vi "AutoDiscardBeads.vi"(10 "Minimum bead validity":dbl=1.0, 11 "Buffer Image":T1) -> ()   [LabVIEW 2011]
uses:
  <vilib>/vision/Image Controls.llb/IMAQ Image.ctl
  GlobalVariables.vi
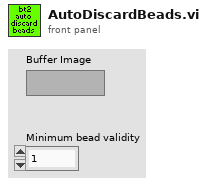
[diagram p1: front panel]
types:
  T1 = typedef "IMAQ Image.ctl" = refnum<image>
  T2 = typedef "MeasureConfigType.ctl" = cluster{"Bead locations":cluster{"X":i32, "Y":i32}[], "ROI":i32, "Experiment base path":path, "Image output subdir":string, "Output mode":T3, "Traces output subdir":string, "QTrk Settings":T4, "Tracking Config":T5, "Experiment Name":string, "Program":T8, "ZLUT":sgl[][][], "Camera settings":T15, "Experiment Script":string, "Max frames in memory":i32, "Save traces as binary":bool, "Pixel Calibration Gain Image":string, "Pixel Calibration Offset Image":string, "Use pixel calibration images":bool, "Internal camera settings":string, "Trace write interval":i32}
  T3 = typedef "MeasureConfigOutputMode.ctl" = enum16{"None", "Track", "SaveImages"}
  T4 = typedef "QTrkSettings.ctl" = cluster{"Image width":i32, "Image height":i32, "Number of threads (CPU based)":i32, "CUDA Device":i32, "COM Background correction factor":sgl, "ZLUT MinRadius":sgl, "ZLUT Radial sample density":sgl, "ZLUT Angular sample density":sgl, "ZLUT ROI Coverage":sgl, "QI Iterations":i32, "QI MinRadius":sgl, "QI Radial sample density":sgl, "QI Angular sample density":sgl, "QI ROI Coverage":sgl, "QI Angular Step \nIteration Factor":sgl, "XCOR Profile Length":i32, "XCOR Profile Width":i32, "XCOR Iterations":i32, "Gaussian 2D Fit Iterations":i32, "Gaussian 2D Sigma (pixels)":sgl, "Downsample":i32}
  T5 = typedef "TrackingConfigType.ctl" = cluster{"Number of steps":i32, "ZLUT stepsize (um)":sgl, "Z correction factor":sgl, "Start piezo Z (um)":sgl, "Pixel size (nm)":sgl, "2D Localization Type":T6, "Z Command (None)":T7, "Z Piezo scale":bool, "ZLUT Building\nimages per frame":i32}
  T6 = typedef "QTrkLocalizationType.ctl" = enum16{"Center-of-Mass", "1D Cross-Correlation", "Quadrant Interpolation", "Gaussian 2D MLE", "QI + ZLUTAlign", "ZLUTAlign", "QI + FourierLUT"}
  T7 = typedef "QTrkZCommandType.ctl" = enum16{"Nothing", "ComputeZ", "BuildRadialZLUT", "BuildImageZLUT", "RadialZLUT+ImageZLUT"}
  T8 = typedef "ExperimentProgramType.ctl" = cluster{"Commands":T9[], "Motor Axis accuracy conditions":T12, "Axis flags":T14}
  T9 = typedef "ExProgCommandType.ctl" = cluster{"cmd":T10, "axis":T11, "value/pos":dbl, "speed":dbl, "name":string}
  T10 = typedef "ExProgCommandEnumType.ctl" = enum16{"wait", "move", "acquire", "idle", "rmove", "when", "section", "stop"}
  T11 = typedef "MotorAxisEnum.ctl" = enum16{"no axis", "magrot", "magpos", "px", "py", "pz", "camx", "camy"}
  T12 = typedef "MotorPosType.ctl" = cluster{"Magnet Z":dbl, "Magnet rotation":dbl, "Camera":T13, "Piezo XY":T13, "Piezo Z":dbl}
  T13 = typedef "XYf.ctl" = cluster{"X":sgl, "Y":sgl}
  T14 = typedef "MotorPosFlagsType.ctl" = cluster{"Magnet Z":bool, "Magnet rotation":bool, "Camera":cluster{"X":bool, "Y":bool}, "Piezo XY":cluster{"X":bool, "Y":bool}, "Piezo Z":bool}
  T15 = typedef "GenericCameraConfigType.ctl" = cluster{"Framerate (Hz)":i32, "Exposure time (us)":i32, "Image size":cluster{"Width":i32, "Height":i32}, "Number of buffers":i32}
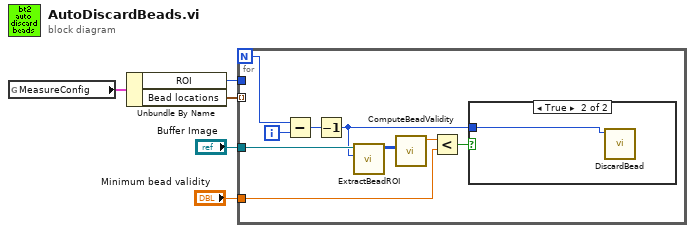
[diagram p0: block diagram]
diagram:
  n1 = global read "GlobalVariables.vi" "MeasureConfig"() -> (w4:T2)
  n2 = Unbundle By Name(w4) -> ("ROI"=w2:i32, "Bead locations"=w3:cluster{"X":i32, "Y":i32}[])
  n3 = for {
    N -> [w12]
    tunnel: "Buffer Image" -> [w14]
    tunnel: w3 -> [_] mode=indexing
    tunnel: w2 -> [_]
    tunnel: "Minimum bead validity" -> [w8]
    i -> [w11]
    n4 = Subtract(x=w12, y=w11) -> (x-y=w10:i32)
    n5 = Decrement(x=w10) -> (x-1=w6:i32)
    n6 = call "ExtractBeadROI.vi"("Bead index"=w6, "Image"=w14) -> ("Image Pixels (U8)"=w13:u8[][])  [unwired: 9 in]
    n7 = call "ComputeBeadValidity.vi"("Image Pixels (U8)"=w13) -> ("Bead validity"=w9:dbl)  [unwired: 10 in]
    n8 = Less?(x=w9, y=w8) -> (x < y?=w7:bool)
    n9 = case shown="True" w7 {
      tunnel: w6 -> [_ w15]
      frame False {
      }
      frame True {
        n10 = call "DiscardBead.vi"("Bead index"=w15) -> ()  [unwired: 11 in]
      }
    }
  }
